vi "Build Command.vi"(8 "error in (no error)":errorcluster, 11 "Console Wrapper in":refnum<class "Console Wrapper.lvclass">) -> (0 "error out":errorcluster, 3 "Console Wrapper out":refnum<class "Console Wrapper.lvclass">)   [LabVIEW 2020, in "Console Wrapper.lvclass"]
doc: "Builds a command to be executed in command line. the structure is as folllows:\n\n[Application] [Command] [Option] [Value] ...\n\nYou can run the command with as much options as you need."
uses:
  Console Wrapper.lvclass
  Console Wrapper.lvclass/Console Wrapper.ctl
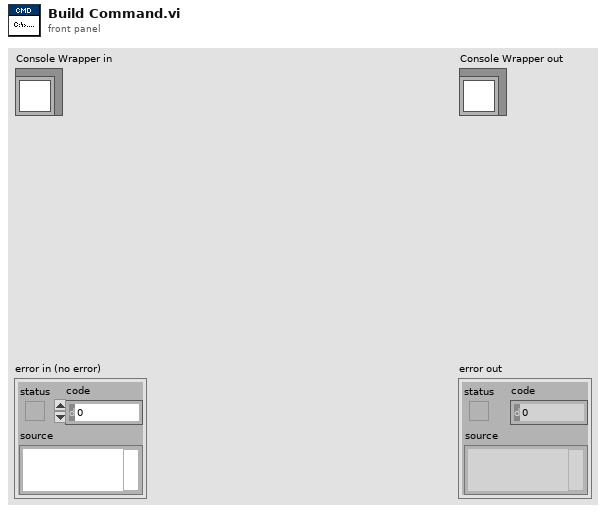
[diagram p1: front panel]
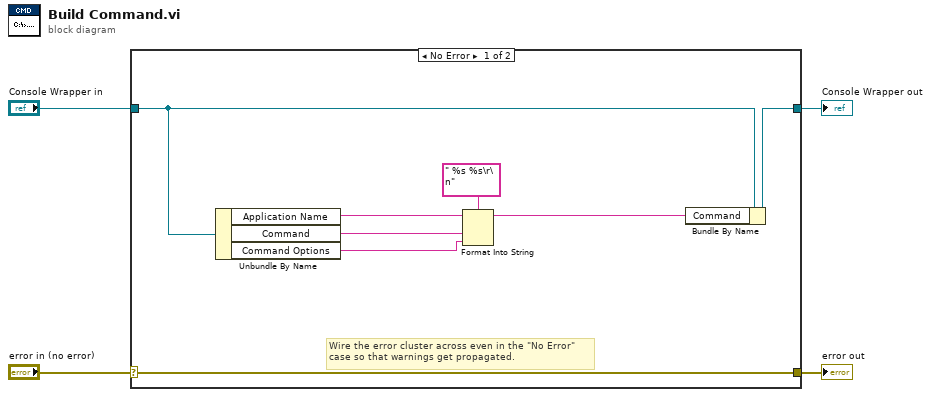
[diagram p0: block diagram]
diagram:
  n1 = case shown="No Error" "error in (no error)" {
    selector: "error in (no error)" -> [w12 w14]
    tunnel: [w12 w14] -> w3
    tunnel: [w9 w13] -> w1
    tunnel: "Console Wrapper in" -> [w10 w13]
    frame No Error {
      # "Wire the error cluster across even in the \"No Error\"\ncase so that warnings get propagated."
      n2 = Unbundle By Name(w10) -> ("Application Name"=w7:string, "Command"=w6:string, "Command Options"=w5:string)
      n3 = Format Into String(format string=" %s %s\r\n", initial string=w7, w6, w5) -> (resulting string=w8:string)  [unwired: 1 in, 1 out]
      n4 = Bundle By Name(cluster=w10, "Command"=w8) -> (w9:refnum<class "Console Wrapper.lvclass">)
    }
    frame Error {
    }
  }
  "error out" <- w3
  "Console Wrapper out" <- w1
